vi "Run Command.vi"(2 "Line Index In":i32, 3 "Script":string) -> (0 "Line Index Out":i32, 1 "Done":bool)   [LabVIEW 2015]
doc: "Looks at a line and runs the appropriate command. Add new commands to this vi."
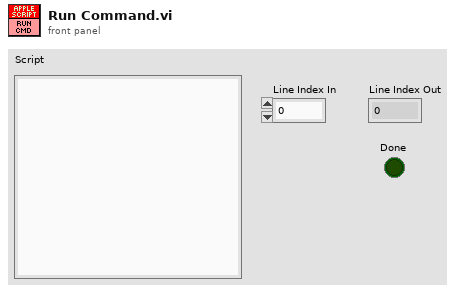
[diagram p1: front panel]
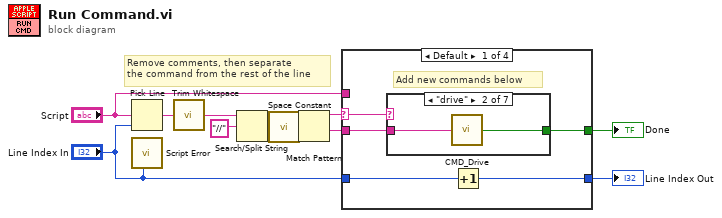
[diagram p0: block diagram]
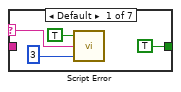
[diagram p2: hidden frame]
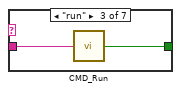
[diagram p3: hidden frame]
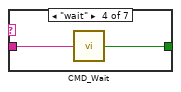
[diagram p4: hidden frame]
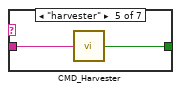
[diagram p5: hidden frame]
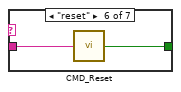
[diagram p6: hidden frame]
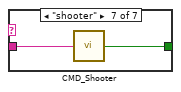
[diagram p7: hidden frame]
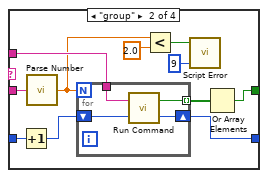
[diagram p8: hidden frame]
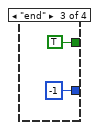
[diagram p9: hidden frame]
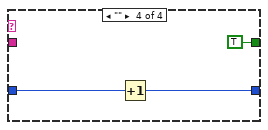
[diagram p10: hidden frame]
diagram:
  # "Remove comments, then separate\nthe command from the rest of the line"
  n1 = Pick Line(multi-line string="Script", line index="Line Index In") -> (output string=w6:string)  [unwired: 1 in]
  n2 = call "Script Error.vi"("Line Number"="Line Index In") -> ()  [unwired: 4 in, 1 out]
  n3 = call <vilib>:"Trim Whitespace.vi"("string"=w6) -> ("trimmed string"=w4:string)  [unwired: 1 in]
  n4 = Search/Split String(string=w4, search string/char (-)="//") -> (substring before match=w3:string)  [unwired: 1 in, 2 out]
  n5 = call <vilib>:"Space Constant.vi"() -> ("String"=w11:string)
  n6 = Match Pattern(string=w3, regular expression=w11) -> (before substring=w2:string, after substring=w1:string)  [unwired: 1 in, 2 out]
  n7 = case shown="Default" w2 {
    selector: w2 -> [w14 _ _ _]
    tunnel: "Script" -> [_ w43 _ _]
    tunnel: "Line Index In" -> [w16 w39 _ w51]
    tunnel: [w13 w41 TRUE ("Running") TRUE ("Running")] -> w9
    tunnel: [w15 w40 -1 ("Line Index Out") w50] -> w8
    tunnel: w1 -> [w12 w33 _ _]
    frame Default {
      # "Add new commands below"
      n8 = case shown="\"drive\"" w14 {
        selector: w14 -> [w17 _ _ _ _ _ _]
        tunnel: [TRUE w22 w23 w26 w28 w30 w31] -> w13
        tunnel: w12 -> [_ w21 w24 w25 w27 w29 w32]
        frame Default {
          n9 = call "Script Error.vi"("Error?"=TRUE, "Error Details"=w17, "Error Code"=3) -> ()  [unwired: 2 in, 1 out]
        }
        frame "drive" {
          n10 = call "CMD_Drive.vi"("Line"=w21) -> ("Done"=w22:bool)
        }
        frame "run" {
          n11 = call "CMD_Run.vi"("Line"=w24) -> ("Done"=w23:bool)
        }
        frame "wait" {
          n12 = call "CMD_Wait.vi"("Line"=w25) -> ("Done"=w26:bool)
        }
        frame "harvester" {
          n13 = call "CMD_Harvester.vi"("Line"=w27) -> ("Done"=w28:bool)
        }
        frame "reset" {
          n14 = call "CMD_Reset.vi"("Line"=w29) -> ("Done"=w30:bool)
        }
        frame "shooter" {
          n15 = call "CMD_Shooter.vi"("Line"=w32) -> ("Done"=w31:bool)
        }
      }
      n16 = Increment(x=w16) -> (x+1=w15:i32)
    }
    frame "group" {
      n17 = Increment(x=w39) -> (x+1=w38:i32)
      n18 = call "Parse Number.vi"("String"=w33) -> ("Number"=w36:dbl)
      n19 = for {
        N: w36 -> [_]
        tunnel: w43 -> [w47]
        tunnel: [w46] -> w42 mode=indexing
        shift-right: [w45] -> w40
        shift-left: w38 -> [w44]
        n20 = call "Run Command.vi"("Line Index In"=w44, "Script"=w47) -> ("Line Index Out"=w45:i32, "Done"=w46:bool)
      }
      n21 = Less?(x=w36, y=2.0) -> (x < y?=w35:bool)
      n22 = call "Script Error.vi"("Error?"=w35, "Error Code"=9) -> ()  [unwired: 3 in, 1 out]
      n23 = Or Array Elements(Boolean array=w42) -> (logical OR=w41:bool)
    }
    frame "end" {
    }
    frame "" {
      n24 = Increment(x=w51) -> (x+1=w50:i32)
    }
  }
  "Line Index Out" <- w8
  "Done" <- w9
